vi "LVClass_WavefrontCorrector Get Actuator Preferences.vi"(0 "WavefrontCorrector in":refnum<class "WavefrontCorrector.lvclass">, 5 "Index of actuator":i32, 11 "error in (no error)":errorcluster) -> (4 "WavefrontCorrector out":refnum<class "WavefrontCorrector.lvclass">, 6 "Wavefront Corrector State":T1, 15 "error out":errorcluster)   [LabVIEW 2020, in "WavefrontCorrector.lvclass"]
doc: "Get preferences of actuator.\n\n<B>correctorIn</B> : WavefrontCorrector object.\n<B>correctorOut</B> : WavefrontCorrector object.\n<B>actuator_index</B> : Index of the actuator.\n<B>min</B> : WavefrontCorrector actuator preferences : lowest command value.\n<B>max</B> : WavefrontCorrector actuator preferences : highest command value.\n<B>validity</B> : WavefrontCorrector actuator preferences : status.\n<B>fixed_values</B> : WavefrontCorrector actuator preferences : fixed positions."
uses:
  WavefrontCorrector.lvclass
  Controls/Wavefront Corrector states - ONE.ctl
  WavefrontCorrector.lvclass/WavefrontCorrector.ctl
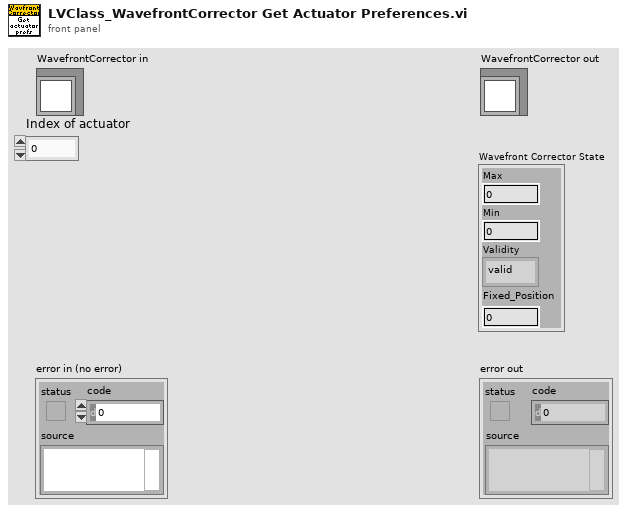
[diagram p1: front panel]
types:
  T1 = typedef "Wavefront Corrector states - ONE.ctl" = cluster{"Max":sgl, "Min":sgl, "Validity":enum16{"valid", "fixed", "invalid"}, "Fixed_Position":sgl}
  T2 = typedef "ClassID.ctl" = i64
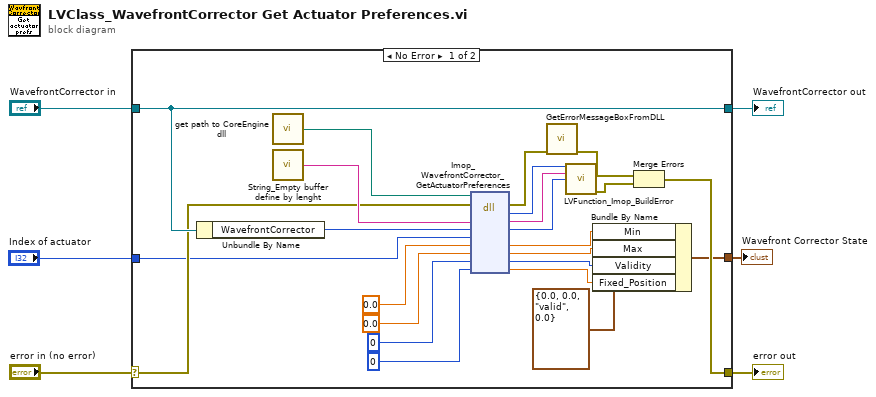
[diagram p0: block diagram]
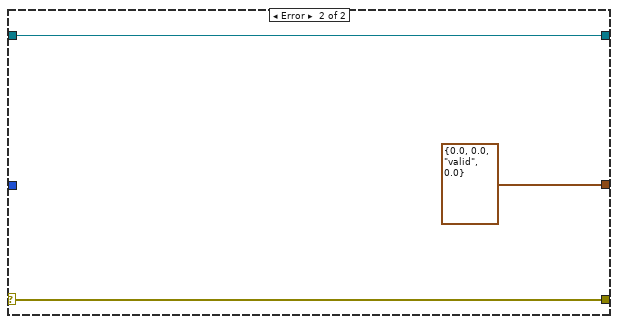
[diagram p2: hidden frame]
diagram:
  n1 = case shown="No Error" "error in (no error)" {
    selector: "error in (no error)" -> [w16 w32]
    tunnel: [w15 w32] -> w5
    tunnel: [w27 w31] -> w3
    tunnel: "WavefrontCorrector in" -> [w27 w31]
    tunnel: [w9 T1 {"Max"=0.0, "Min"=0.0, "Validity"=enum."valid", "Fixed_Position"=0.0} ("Actuator state")] -> w2
    tunnel: "Index of actuator" -> [w8 _]
    frame No Error {
      n2 = Unbundle By Name(w27) -> ("WavefrontCorrector"=w26:T2)
      n3 = call "get path to CoreEngine dll.vi"() -> ("path to wavekit library"=w29:path)  [unwired: 14 in, 1 out]
      n4 = call "String_Empty buffer define by lenght.vi"() -> ("Empty buffer"=w28:string)  [unwired: 1 in]
      n5 = dll-call lib="D:/FLE/0.Code/CoreEngine4_Suite/LV2011_interface/DLLs/c_interface_vc100.dll" fn="Imop_WavefrontCorrector_GetActuatorPreferences"(path in=w29, error in=w16, "Message"=w28, "Wavefront Corrector"=w26, "Index of actuator"=w8, "Min"=sgl 0.0, "Max"=sgl 0.0, "Validity"=0, "Fixed_positions"=0) -> (error out=w21:errorcluster, "return type"=w19:i32, "Message"=w18:string, "Wavefront Corrector"=w7:i64, "Min"=w13:sgl, "Max"=w12:sgl, "Validity"=w11:i32, "Fixed_positions"=w10:sgl)  [unwired: 2 in, 1 out]
      n6 = call "GetErrorMessageBoxFromDLL.vi"("error IN"=w21) -> ("error OUT"=w20:errorcluster)  [unwired: 10 in]
      n7 = call "LVFunction_Imop_BuildError.vi"("code"=w19, "String to Prepend to source (\"\")"=w18, "Adresse"=w7) -> ("error out"=w17:errorcluster)  [unwired: 12 in]
      n8 = Bundle By Name(cluster=T1 {"Max"=0.0, "Min"=0.0, "Validity"=enum."valid", "Fixed_Position"=0.0} ("Actuator state"), "Min"=w13, "Max"=w12, "Validity"=w11, "Fixed_Position"=w10) -> (w9:T1)
      n9 = Merge Errors(w20, w17) -> (w15:errorcluster)
    }
    frame Error {
    }
  }
  "error out" <- w5
  "WavefrontCorrector out" <- w3
  "Wavefront Corrector State" <- w2
